vi "Host Pilot Access (SubVI).vi"(8 "error in":errorcluster, 11 "Master":bool) -> (0 "error out":errorcluster)   [LabVIEW 2021]
doc: "This vi is used as global variable the Access Status passing to the UDP transfer loop . The boolean status is converted in to 1/0 ."
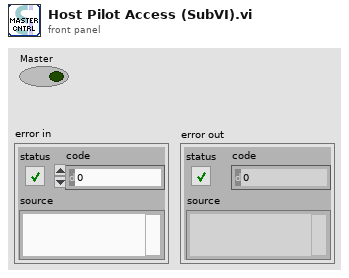
[diagram p1: front panel]
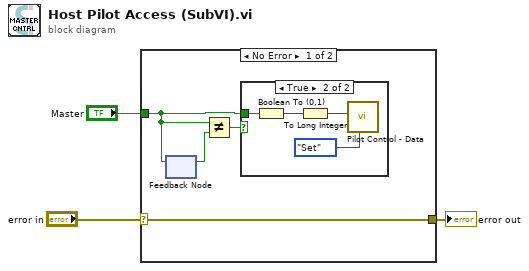
[diagram p0: block diagram]
diagram:
  n1 = case shown="No Error" "error in" {
    selector: "error in" -> [w4 w12]
    tunnel: "Master" -> [w7 _]
    tunnel: [w4 w12] -> w1
    frame No Error {
      n2 = feedback #1() -> (w5:bool)  [unwired: 1 in]
      n3 = feedback-in #1(w7) -> ()
      n4 = Not Equal?(x=w7, y=w5) -> (x != y?=w6:bool)
      n5 = case shown="True" w6 {
        tunnel: w7 -> [_ w10]
        frame False {
        }
        frame True {
          n6 = Boolean To (0,1)(Boolean=w10) -> (0, 1=w8:i16)
          n7 = To Long Integer(number=w8) -> (32bit integer=w9:i32)
          n8 = call "Pilot Control - Data.vi"("Operation"=enum16{"Init", "Get", "Set"}."Set", "Data in"=w9) -> ()  [unwired: 9 in, 1 out]
        }
      }
    }
    frame Error {
    }
  }
  "error out" <- w1
